vi "Set gRPC ID.vi"(10 "gRPC ID":T1, 11 "OOP Server in":refnum<class "Servicer.lvclass">) -> (3 "OOP Server out":refnum<class "Servicer.lvclass">)   [LabVIEW 2019]
uses:
  Servicer.lvclass/Servicer.ctl
  Servicer.lvclass
  gRPC lv Support/grpc-lvsupport/grpcId.ctl
  gRPC lv Support/grpc-lvsupport/grpc-lvsupport.lvlib
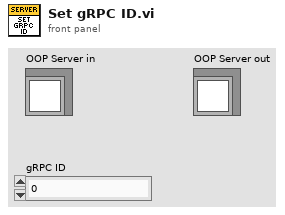
[diagram p1: front panel]
types:
  T1 = typedef "grpc-lvsupport.lvlib/grpcId.ctl" = u64
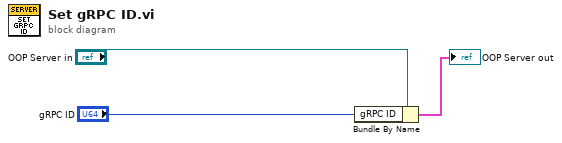
[diagram p0: block diagram]
diagram:
  n1 = Bundle By Name(cluster="OOP Server in", "gRPC ID"="gRPC ID") -> (→"OOP Server out":cluster{})
